vi "svl_Design HighPass Filter.vi"(6 "highpass filter order":i32, 7 "filter design method":enum16{"Elliptic", "Butterworth"}(ring), 8 "error in (no error)":errorcluster, 9 "highpass cutoff frequency":dbl format="%.2f", 11 "dt":dbl) -> (0 "error out":errorcluster, 2 "IIR Filter Cluster":T1 {"Forward Coefficients" format="%.2f"; "Reverse Coefficients" format="%.2f"})   [LabVIEW 2017, in "SoundVib_Integration.lvlib"]
uses:
  <vilib>/addons/Sound and Vibration/svt_Integration/SoundVib_Integration.lvlib
  <vilib>/Analysis/3filter.llb/Filter Passband Type.ctl
  <vilib>/Analysis/NI_AALBase.lvlib
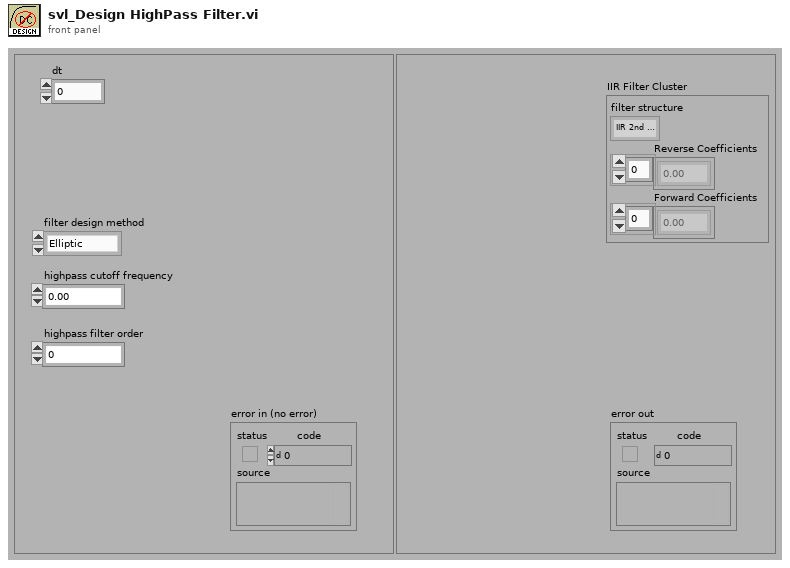
[diagram p1: front panel]
types:
  T1 = cluster{"filter structure":enum32{"IIR 2nd Order", "IIR 4th Order"}, "Reverse Coefficients":dbl[], "Forward Coefficients":dbl[]}
  T2 = typedef "NI_AALBase.lvlib/Filter Passband Type.ctl" = enum32{"Lowpass", "Highpass", "Bandpass", "Bandstop"}
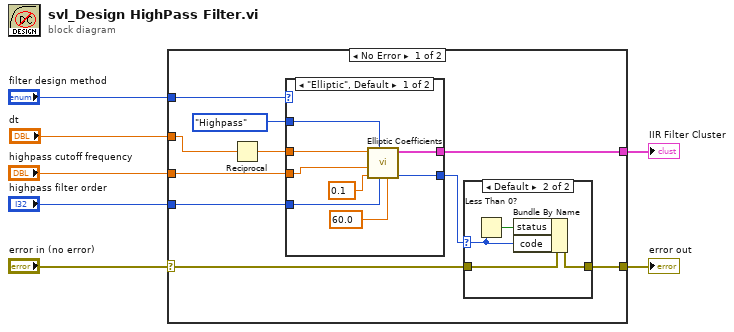
[diagram p0: block diagram]
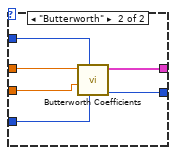
[diagram p2: hidden frame]
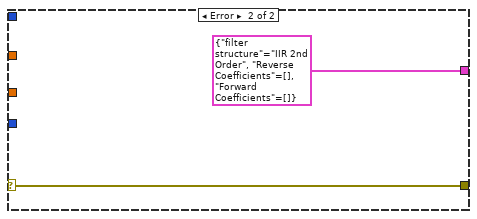
[diagram p4: hidden frame]
diagram:
  n1 = case shown="No Error" "error in (no error)" {
    selector: "error in (no error)" -> [w15 w38]
    tunnel: "highpass cutoff frequency" -> [w17 _]
    tunnel: "highpass filter order" -> [w16 _]
    tunnel: [w14 w38] -> w6
    tunnel: [w12 T1 {"filter structure"=enum."IIR 2nd Order", "Reverse Coefficients"=[], "Forward Coefficients"=[]} ("IIR Filter Cluster")] -> w7
    tunnel: "dt" -> [w9 _]
    tunnel: "filter design method" -> [w10 _]
    frame No Error {
      n2 = Reciprocal(x=w9) -> (1/x=w8:dbl)
      n3 = case shown="\"Elliptic\", Default" w10 {
        tunnel: w17 -> [w20 w31]
        tunnel: w16 -> [w22 w30]
        tunnel: [w18 w29] -> w13
        tunnel: [w19 w28] -> w12
        tunnel: w8 -> [w21 w26]
        tunnel: Filter_Passband_Type."Highpass" ("filter type") -> [w23 w27]
        frame "Elliptic", Default {
          n4 = call <vilib>:"Elliptic Coefficients.vi"("stopband attenuation (dB)"=60.0, "order"=w22, "filter type"=w23, "passband ripple (dB)"=0.1, "low cutoff freq: fl"=w20, "sampling freq: fs"=w21) -> ("error"=w18:i32, "IIR Filter Cluster"=w19:T1)  [unwired: 4 in]
        }
        frame "Butterworth" {
          n5 = call <vilib>:"Butterworth Coefficients.vi"("order"=w30, "filter type"=w27, "low cutoff freq: fl"=w31, "sampling freq: fs"=w26) -> ("error"=w29:i32, "IIR Filter Cluster"=w28:T1)  [unwired: 6 in]
        }
      }
      n6 = case shown="Default" w13 {
        selector: w13 -> [_ w34]
        tunnel: w15 -> [w32 w36]
        tunnel: [w32 w35] -> w14
        frame 0 {
        }
        frame Default {
          n7 = Less Than 0?(x=w34) -> (x < 0?=w33:bool)
          n8 = Bundle By Name(cluster=w36, "status"=w33, "code"=w34) -> (w35:errorcluster)
        }
      }
    }
    frame Error {
    }
  }
  "IIR Filter Cluster" <- w7
  "error out" <- w6
